vi "Global 1.vi"() -> ()   [LabVIEW 2012]
panel:
  out "AMCS_Data":i32[][](array[numeric])
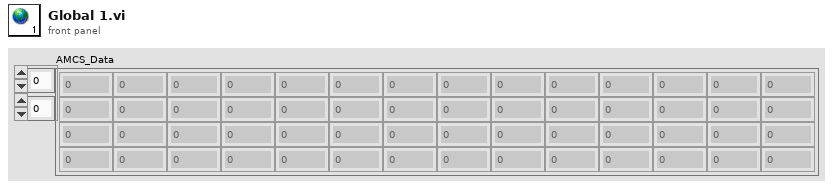
[diagram p1: front panel]
diagram:
